vi "Fetch Multi Eval Meas List MERR RMS Results.vi"(6 "Window Position (Low)":i32(ring) items=["Low", "High"], 8 "error in (no error)":errorcluster, 9 "Result Type (Current)":i32(ring) items=["Current", "Average", "Extreme", "Standard Deviation"], 10 "Instance (1)":T1=1, 11 "VISA resource name":refnum<visa-resource-name>) -> (0 "error out":errorcluster, 1 "Results":dbl[](array[numeric]) format="%^.3e", 2 "Reliability":i32, 3 "VISA resource name out":refnum<visa-resource-name>)   [LabVIEW 2020, in "Rohde&Schwarz CMWXP NR FR1 Measurement.lvlib"]
doc: "Return magnitude error RMS values for low and high EVM window position, for all measured list mode segments.\n\nAttributes:\nRSCMWXPNRFR1M_ATTR_FETCH_MULTI_EVAL_MEAS_LIST_MERR_RMS_LOW_CURRENT_RESULTS\nRSCMWXPNRFR1M_ATTR_FETCH_MULTI_EVAL_MEAS_LIST_MERR_RMS_LOW_AVERAGE_RESULTS\nRSCMWXPNRFR1M_ATTR_FETCH_MULTI_EVAL_MEAS_LIST_MERR_RMS_LOW_EXTREME_RESULTS\nRSCMWXPNRFR1M_ATTR_FETCH_MULTI_EVAL_MEAS_LIST_MERR_RMS_LOW_STANDARD_DEVIATION_RESULTS\nRSCMWXPNRFR1M_ATTR_FETCH_MULTI_EVAL_MEAS_LIST_MERR_RMS_HIGH_CURRENT_RESULTS\nRSCMWXPNRFR1M_ATTR_FETCH_MULTI_EVAL_MEAS_LIST_MERR_RMS_HIGH_AVERAGE_RESULTS\nRSCMWXPNRFR1M_ATTR_FETCH_MULTI_EVAL_MEAS_LIST_MERR_RMS_HIGH_EXTREME_RESULTS\nRSCMWXPNRFR1M_ATTR_FETCH_MULTI_EVAL_MEAS_LIST_MERR_RMS_HIGH_STANDARD_DEVIATION_RESULTS\n\nRemote-control commands:\nFETCh:NRSub:MEAS<i>:MEValuation:LIST:MODulation:MERRor:RMS:LOW:CURRent?\nFETCh:NRSub:MEAS<i>:MEValuation:LIST:MODulation:MERRor:RMS:LOW:AVERage?\nFETCh:NRSub:MEAS<i>:MEValuation:LIST:MODulation:MERRor:RMS:LOW:EXTReme?\nFETCh:NRSub:MEAS<i>:MEValuation:LIST:MODulation:MERRor:RMS:LOW:SDEViation?\nFETCh:NRSub:MEAS<i>:MEValuation:LIST:MODulation:MERRor:RMS:HIGH:CURRent?\nFETCh:NRSub:MEAS<i>:MEValuation:LIST:MODulation:MERRor:RMS:HIGH:AVERage?\nFETCh:NRSub:MEAS<i>:MEValuation:LIST:MODulation:MERRor:RMS:HIGH:EXTReme?\nFETCh:NRSub:MEAS<i>:MEValuation:LIST:MODulation:MERRor:RMS:HIGH:SDEViation?"
uses:
  <instrlib>/Rohde&Schwarz CMWXP NR FR1 Measurement/Rohde&Schwarz CMWXP NR FR1 Measurement.lvlib
  <instrlib>/Rohde&Schwarz CMWXP NR FR1 Measurement/Private/_Instance.ctl
  <instrlib>/Rohde&Schwarz CMWXP NR FR1 Measurement/Private/rsidr_core.llb/rsidr_core.lvlib
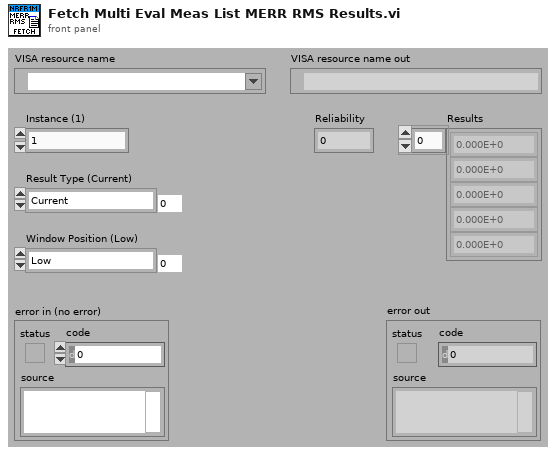
[diagram p1: front panel]
types:
  T1 = typedef "Rohde&Schwarz CMWXP NR FR1 Measurement.lvlib/_Instance.ctl" = i32
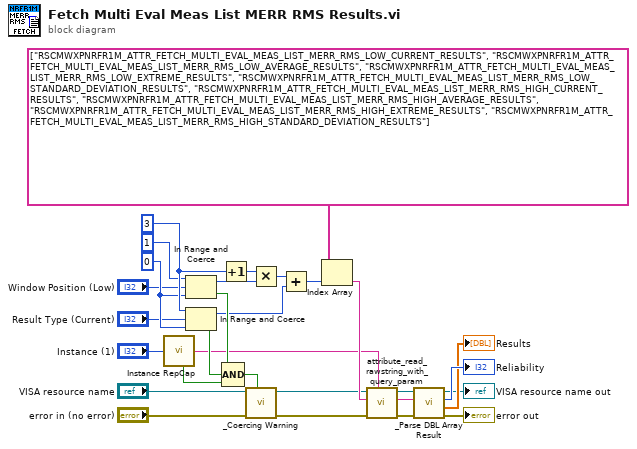
[diagram p0: block diagram]
diagram:
  w25 = 3
  w24 = 0
  n1 = call <instrlib>:"Instance RepCap.vi"("Instance In"="Instance (1)") -> ("In Range?"=w27:bool, "RepCap Identifier Out"=w13:string)  [unwired: 1 in]
  n2 = In Range and Coerce(upper limit=1, x="Window Position (Low)", lower limit=w24) -> (coerced(x)=w20:i32, In Range?=w21:bool)
  n3 = In Range and Coerce(upper limit=w25, x="Result Type (Current)", lower limit=w24) -> (coerced(x)=w19:i32, In Range?=w22:bool)
  n4 = Increment(x=w25) -> (x+1=w26:i32)
  n5 = Compound Arithmetic op=AND(w21, w22, w27) -> (w28:bool)
  n6 = call <instrlib>:"_Coercing Warning.vi"("In Range?"=w28, "error in (no error)"="error in (no error)", "VISA resource name"="VISA resource name") -> ("error out"=w14:errorcluster, "VISA resource name out"=w15:refnum<visa-resource-name>)  [unwired: 7 in]
  n7 = Multiply(x=w26, y=w20) -> (x*y=w29:i32)
  n8 = Add(x=w29, y=w19) -> (x+y=w18:i32)
  n9 = Index Array(array=string[] ["RSCMWXPNRFR1M_ATTR_FETCH_MULTI_EVAL_MEAS_LIST_MERR_RMS_LOW_CURRENT_RESULTS", "RSCMWXPNRFR1M_ATTR_FETCH_MULTI_EVAL_MEAS_LIST_MERR_RMS_LOW_AVERAGE_RESULTS", "RSCMWXPNRFR1M_ATTR_FETCH_MULTI_EVAL_MEAS_LIST_MERR_RMS_LOW_EXTREME_RESULTS", "RSCMWXPNRFR1M_ATTR_FETCH_MULTI_EVAL_MEAS_LIST_MERR_RMS_LOW_STANDARD_DEVIATION_RESULTS", "RSCMWXPNRFR1M_ATTR_FETCH_MULTI_EVAL_MEAS_LIST_MERR_RMS_HIGH_CURRENT_RESULTS", "RSCMWXPNRFR1M_ATTR_FETCH_MULTI_EVAL_MEAS_LIST_MERR_RMS_HIGH_AVERAGE_RESULTS", "RSCMWXPNRFR1M_ATTR_FETCH_MULTI_EVAL_MEAS_LIST_MERR_RMS_HIGH_EXTREME_RESULTS", "RSCMWXPNRFR1M_ATTR_FETCH_MULTI_EVAL_MEAS_LIST_MERR_RMS_HIGH_STANDARD_DEVIATION_RESULTS"], index=w18) -> (element=w16:string)
  n10 = call <instrlib>:"attribute_read_rawstring_with_query_param.vi"("Repeated Capability"=w13, "error in"=w14, "Attribute ID"=w16, "VISA resource name"=w15) -> ("error out"=w12:errorcluster, "Raw String out"=w11:string, "VISA resource name out"=w10:refnum<visa-resource-name>)  [unwired: 5 in]
  n11 = call <instrlib>:"_Parse DBL Array Result.vi"("error in (no error)"=w12, "Input String"=w11, "VISA resource name"=w10) -> ("error out"=→"error out":errorcluster, "Results"=→"Results":dbl[], "Reliability"=→"Reliability":i32, "VISA resource name out"=→"VISA resource name out":refnum<visa-resource-name>)  [unwired: 5 in]
